vi "Read SH-Persis.vi"(8 "error in (no error)":errorcluster, 11 "Power Supply in":refnum<class "Power Supply.lvclass">) -> (0 "error out":errorcluster, 1 "SHon?":bool, 2 "pers?":bool, 3 "Power Supply out":refnum<class "Power Supply.lvclass">, 4 "Switch Heater":T2={"Value"=1, "Off (at zero field)"=FALSE, "On"=TRUE, "Off (at field)"=FALSE, "No switch fitted"=FALSE, "Confirm"=FALSE}, 5 "SHstatus":T1)   [LabVIEW 2009, in "Power Supply.lvclass"]
uses:
  Power Supply.lvclass
  Switch Heater Status.ctl
  Power Supply.lvclass/Power Supply.ctl
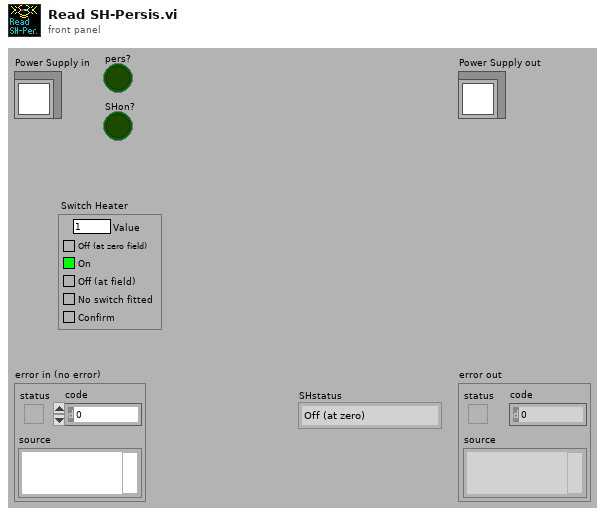
[diagram p1: front panel]
types:
  T1 = typedef "Power Supply.lvclass/Switch Heater Status.ctl" = enum16{"Off (at zero)", "On", "Off (at field)", "Other"}
  T2 = cluster{"Value":i16, "Off (at zero field)":bool, "On":bool, "Off (at field)":bool, "No switch fitted":bool, "Confirm":bool}
  T3 = typedef "OxfordAddress.ctl" = cluster{"Com Port":i32, "ISOBUS Address":i32, "GPIB Address":i16, "Communication":enum16{"RS232", "ISOBUS", "GPIB", "Gateway"}}
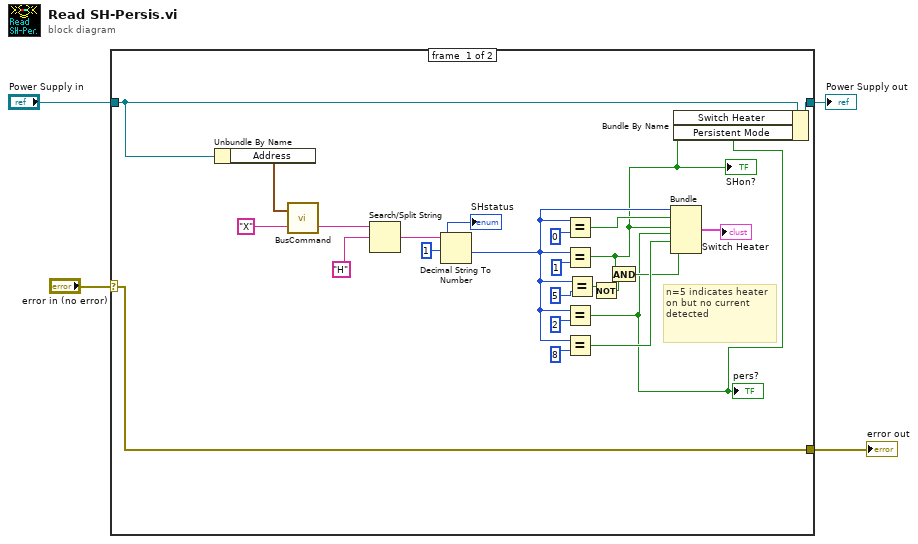
[diagram p0: block diagram]
diagram:
  n1 = case shown="No Error" "error in (no error)" {
    selector: "error in (no error)" -> [w9 w28]
    tunnel: "Power Supply in" -> [w10 w29]
    tunnel: [w8 w29] -> w4
    tunnel: [w9 w28] -> w2
    frame #0 {
      # "n=5 indicates heater on but no current detected"
      n2 = Unbundle By Name(w10) -> ("Address"=w14:T3)
      n3 = call "BusCommand.vi"("Command"="X", "Instrument address (in)"=w14) -> ("Reply"=w19:string)  [unwired: 1 out]
      n4 = Search/Split String(string=w19, search string/char (-)="H") -> (match + rest of string=w26:string)  [unwired: 3 out]
      n5 = Decimal String To Number(string=w26, offset=1) -> (number=w11:i32)  [unwired: 2 out]
      "SHstatus" <- w11
      n6 = Equal?(x=w11, y=0) -> (x = y?=w23:bool)
      n7 = Equal?(x=w11, y=1) -> (x = y?=w6:bool)
      "SHon?" <- w6
      n8 = Equal?(x=w11, y=2) -> (x = y?=w5:bool)
      "pers?" <- w5
      n9 = Equal?(x=w11, y=8) -> (x = y?=w20:bool)
      n10 = Equal?(x=w11, y=5) -> (x = y?=w15:bool)
      n11 = Not(x=w15) -> (.not. x?=w16:bool)
      n12 = And(x=w6, y=w16) -> (x .and. y?=w18:bool)
      n13 = Bundle(w11, w23, w6, w5, w20, w18) -> (→"Switch Heater":cluster{i32, bool, bool, bool, bool, bool})  [unwired: 1 out]
      n14 = Bundle By Name(cluster=w10, "Switch Heater"=w6, "Persistent Mode"=w5) -> (w8:refnum<class "Power Supply.lvclass">)
    }
    frame #1 {
    }
  }
  "error out" <- w2
  "Power Supply out" <- w4
